vi "Close.vi"(8 "error in (no error)":errorcluster, 11 "uService Template in":refnum<class "TCP Listener.lvclass">) -> (0 "error out":errorcluster, 3 "uService Template out":refnum<class "TCP Listener.lvclass">)   [LabVIEW 2026, in "TALOS.lvlib" / "TCP Listener.lvlib" / "TCP Listener.lvclass"]
uses:
  TCP Listener.lvclass
  Father of all uServices/Father of all uServices/Father of all uServices.lvclass
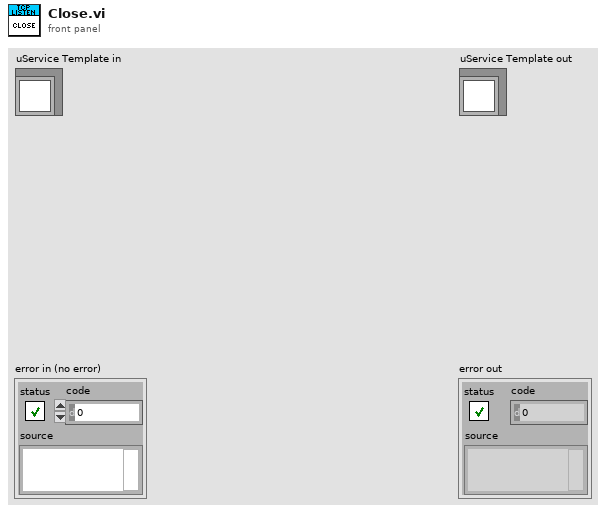
[diagram p1: front panel]
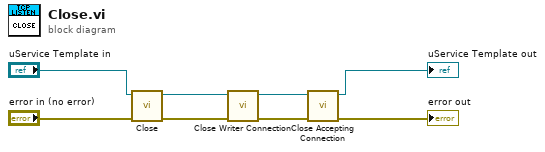
[diagram p0: block diagram]
diagram:
  n1 = call-parent "Close.vi"("error in (no error)"="error in (no error)", "uService Template in"="uService Template in") -> ("error out"=w5:errorcluster, "uService Template out"=w6:refnum<class "TCP Listener.lvclass">)  [unwired: 8 in]
  n2 = call-dynamic "Close Writer Connection.vi"("error in"=w5, "uService Template in"=w6) -> ("error out"=w3:errorcluster, "uService Template out"=w4:refnum<class "TCP Listener.lvclass">)  [unwired: 8 in]
  n3 = call-dynamic "Close Accepting Connection.vi"("error in"=w3, "uService Template in"=w4) -> ("error out"=→"error out":errorcluster, "uService Template out"=→"uService Template out":refnum<class "TCP Listener.lvclass">)  [unwired: 8 in]
